vi "MultiprogrammerConfig.vi"() -> ()   [LabVIEW 2011]
uses:
  editor_lib/Flow_Globals.vi
  Relays.vi
panel:
  in  "H2 Dilute Relay Card":u16(ring)=10 caption="Relay Card" items=["1", "2", "3", "4", "5"]
  in  "Run Relay":u16(ring)=10 caption="Relay" items=["1", "2", "3", "4", "5"]
  in  "Run Relay Card":u16(ring)=10 caption="Relay Card" items=["1", "2", "3", "4", "5"]
  in  "Bubbler In Relay":u16(ring)=10 caption="Relay" items=["1", "2", "3", "4", "5"]
  in  "Bubbler In Relay Card":u16(ring)=10 caption="Relay Card" items=["1", "2", "3", "4", "5"]
  in  "Ga Active Relay":u16(ring)=10 caption="Relay" items=["1", "2", "3", "4", "5"]
  in  "Active Relay Card":u16(ring)=10 caption="Relay Card" items=["1", "2", "3", "4", "5"]
  in  "Ga Remote Relay":u16(ring)=10 caption="Relay" items=["1", "2", "3", "4", "5"]
  in  "Remote Relay Card":u16(ring)=10 caption="Relay Card" items=["1", "2", "3", "4", "5"]
  # "Remote:"
  # "Active:"
  # "Bubbler In:"
  # "Run:"
  # "H2 Dilute"
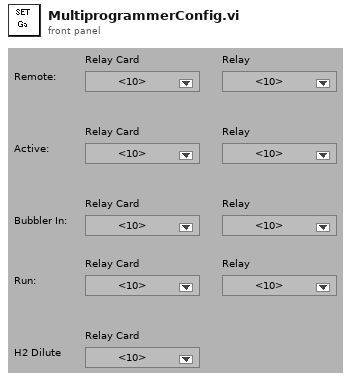
[diagram p1: front panel]
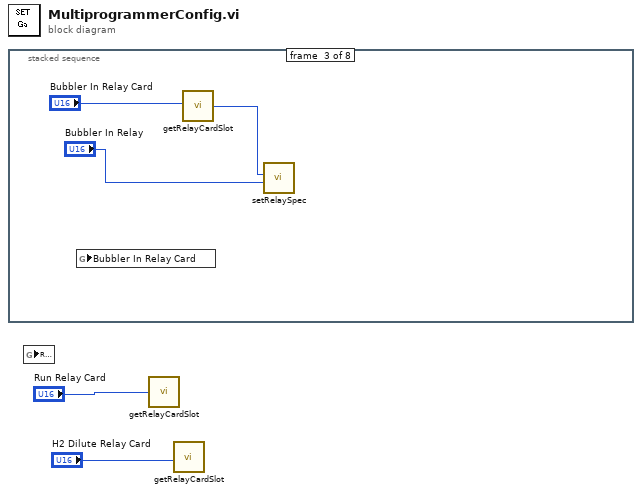
[diagram p0: block diagram]
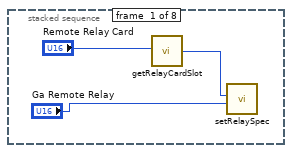
[diagram p2: hidden frame]
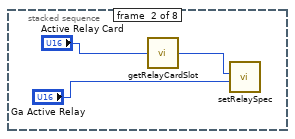
[diagram p3: hidden frame]
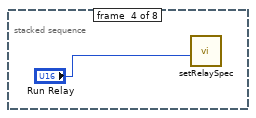
[diagram p4: hidden frame]
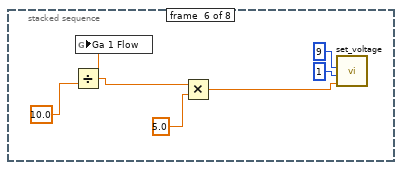
[diagram p6: hidden frame]
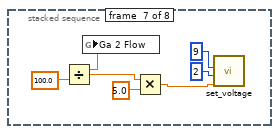
[diagram p7: hidden frame]
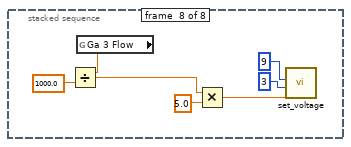
[diagram p8: hidden frame]
diagram:
  n1 = stacked-sequence {
    frame #0 {
      n2 = call "getRelayCardSlot.vi"("Relay Card #"="Remote Relay Card") -> ("Slot"=w3:u16)
      n3 = call "setRelaySpec.vi"("Card"=w3, "Relay"="Ga Remote Relay") -> ("Relay Status"=w6:bool)  [unwired: 1 in, 2 out]
    }
    frame #1 {
      n4 = call "getRelayCardSlot.vi"("Relay Card #"="Active Relay Card") -> ("Slot"=w7:u16)
      n5 = call "setRelaySpec.vi"("Card"=w7, "Relay"="Ga Active Relay") -> ("Relay Status"=w10:bool)  [unwired: 3 out]
    }
    frame #2 {
      n6 = global read "Relays.vi" "Bubbler In Relay Card"() -> ()  [unwired: 1 in]
      n7 = call "getRelayCardSlot.vi"("Relay Card #"="Bubbler In Relay Card") -> ("Slot"=w12:u16)
      n8 = call "setRelaySpec.vi"("Card"=w12, "Relay"="Bubbler In Relay") -> ("Relay Status"=w14:bool)  [unwired: 3 out]
    }
    frame #3 {
      n9 = call "setRelaySpec.vi"("Relay"="Run Relay") -> ("Relay Status"=w16:bool)  [unwired: 1 in, 3 out]
    }
    frame #4 {
    }
    frame #5 {
      n10 = Divide(y=10.0) -> (x=w17:dbl, x/y=w20:dbl)
      n11 = global write "Flow_Globals.vi" "Ga 1 Flow"(w17) -> ()
      n12 = Multiply(x=w20, y=5.0) -> (x*y=w18:dbl)
      n13 = call "set_voltage.vi"("Voltage"=w18, "Channel"=1, "Slot"=9) -> ()  [unwired: 1 in, 1 out]
    }
    frame #6 {
      n14 = Divide(y=100.0) -> (x=w24:dbl, x/y=w26:dbl)
      n15 = global write "Flow_Globals.vi" "Ga 2 Flow"(w24) -> ()
      n16 = Multiply(x=w26, y=5.0) -> (x*y=w25:dbl)
      n17 = call "set_voltage.vi"("Voltage"=w25, "Channel"=2, "Slot"=9) -> ()  [unwired: 1 in, 1 out]
    }
    frame #7 {
      n18 = global read "Flow_Globals.vi" "Ga 3 Flow"() -> (w31:dbl)
      n19 = Divide(x=w31, y=1000.0) -> (x/y=w33:dbl)
      n20 = Multiply(x=w33, y=5.0) -> (x*y=w32:dbl)
      n21 = call "set_voltage.vi"("Voltage"=w32, "Channel"=3, "Slot"=9) -> ()  [unwired: 1 in, 1 out]
    }
  }
  n22 = global read "Relays.vi" item#-1() -> ()  [unwired: 1 in]
  n23 = call "getRelayCardSlot.vi"("Relay Card #"="Run Relay Card") -> ()  [unwired: 1 out]
  n24 = call "getRelayCardSlot.vi"("Relay Card #"="H2 Dilute Relay Card") -> ()  [unwired: 1 out]
